vi "Memory.Array.Subset Reference.vi"(7 "length (-1: rest)":i64=-1 format="%d bytes", 8 "error in (no error)":errorcluster, 9 "index (0)":u64, 11 "Array in":refnum<class "Memory.Array.Void.lvclass">) -> (0 "error out":errorcluster, 2 "subset Array":refnum<class "Memory.Array.Void.lvclass">, 3 "Array out":refnum<class "Memory.Array.Void.lvclass">)   [LabVIEW 2016, in "LabVIEW Memory Manager.lvlib" / "Memory.Array.Void.lvclass"]
uses:
  Memory.Array.Void.lvclass
  Memory.Array.Get Number of Elements.vi
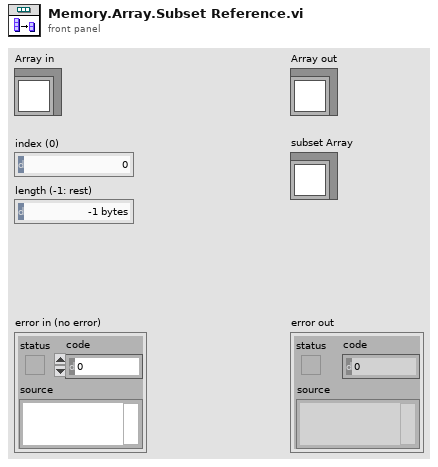
[diagram p1: front panel]
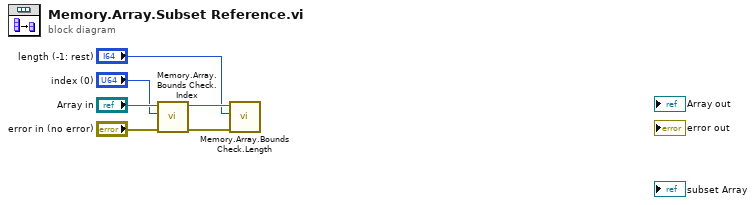
[diagram p0: block diagram]
diagram:
  n1 = call "Memory.Array.Bounds Check.Index.vi"("error in (no error)"="error in (no error)", "index"="index (0)", "Array in"="Array in") -> ("error out"=w3:errorcluster, "Array out"=w4:refnum<class "Memory.Array.Void.lvclass">)  [unwired: 5 in, 2 out]
  n2 = call "Memory.Array.Bounds Check.Length.vi"("error in (no error)"=w3, "length"="length (-1: rest)", "Array in"=w4) -> ()  [unwired: 5 in, 4 out]
